vi "Create Connect Messages.vi"(8 "error in (no error)":errorcluster, 11 "Engine Data in":T2) -> (0 "error out":errorcluster, 1 "Connect Messages":T1[](array[typedef]), 2 "Disconnect Messages":T1[](array[typedef]), 3 "Engine Data out":T2)   [LabVIEW 2017, in "Routing and Faulting Engine.lvlib"]
uses:
  Routing and Faulting Engine.lvlib
  Engine Data.ctl
  Includes/CDMessaging.lvlibp/Producer/Abstract Producer/Abstract Producer.lvclass
  Shared/Compiled.Settings.ctl
  Shared/Communication Configuration.ctl
  Shared/Routing and Faulting Configuration.ctl
  Shared/Routing Channel Configuration.ctl
  Shared/Value-Connections Map.ctl
  Shared/Connection.ctl
  Shared/Alias Mapping.ctl
  Shared/FIFO Indices.ctl
  Device Inputs.ctl
  Device Outputs.ctl
  Producer Message.ctl
  Includes/CDMessaging.lvlibp/Message/Abstract Message/Abstract Message.lvclass
  f117cfd3-3adc-40fc-b63f-36de5ebdde45.vi
  3305a376-d4c0-444a-b726-8088d0367693.vi
  Shared/Routing and Faulting Shared.lvlib
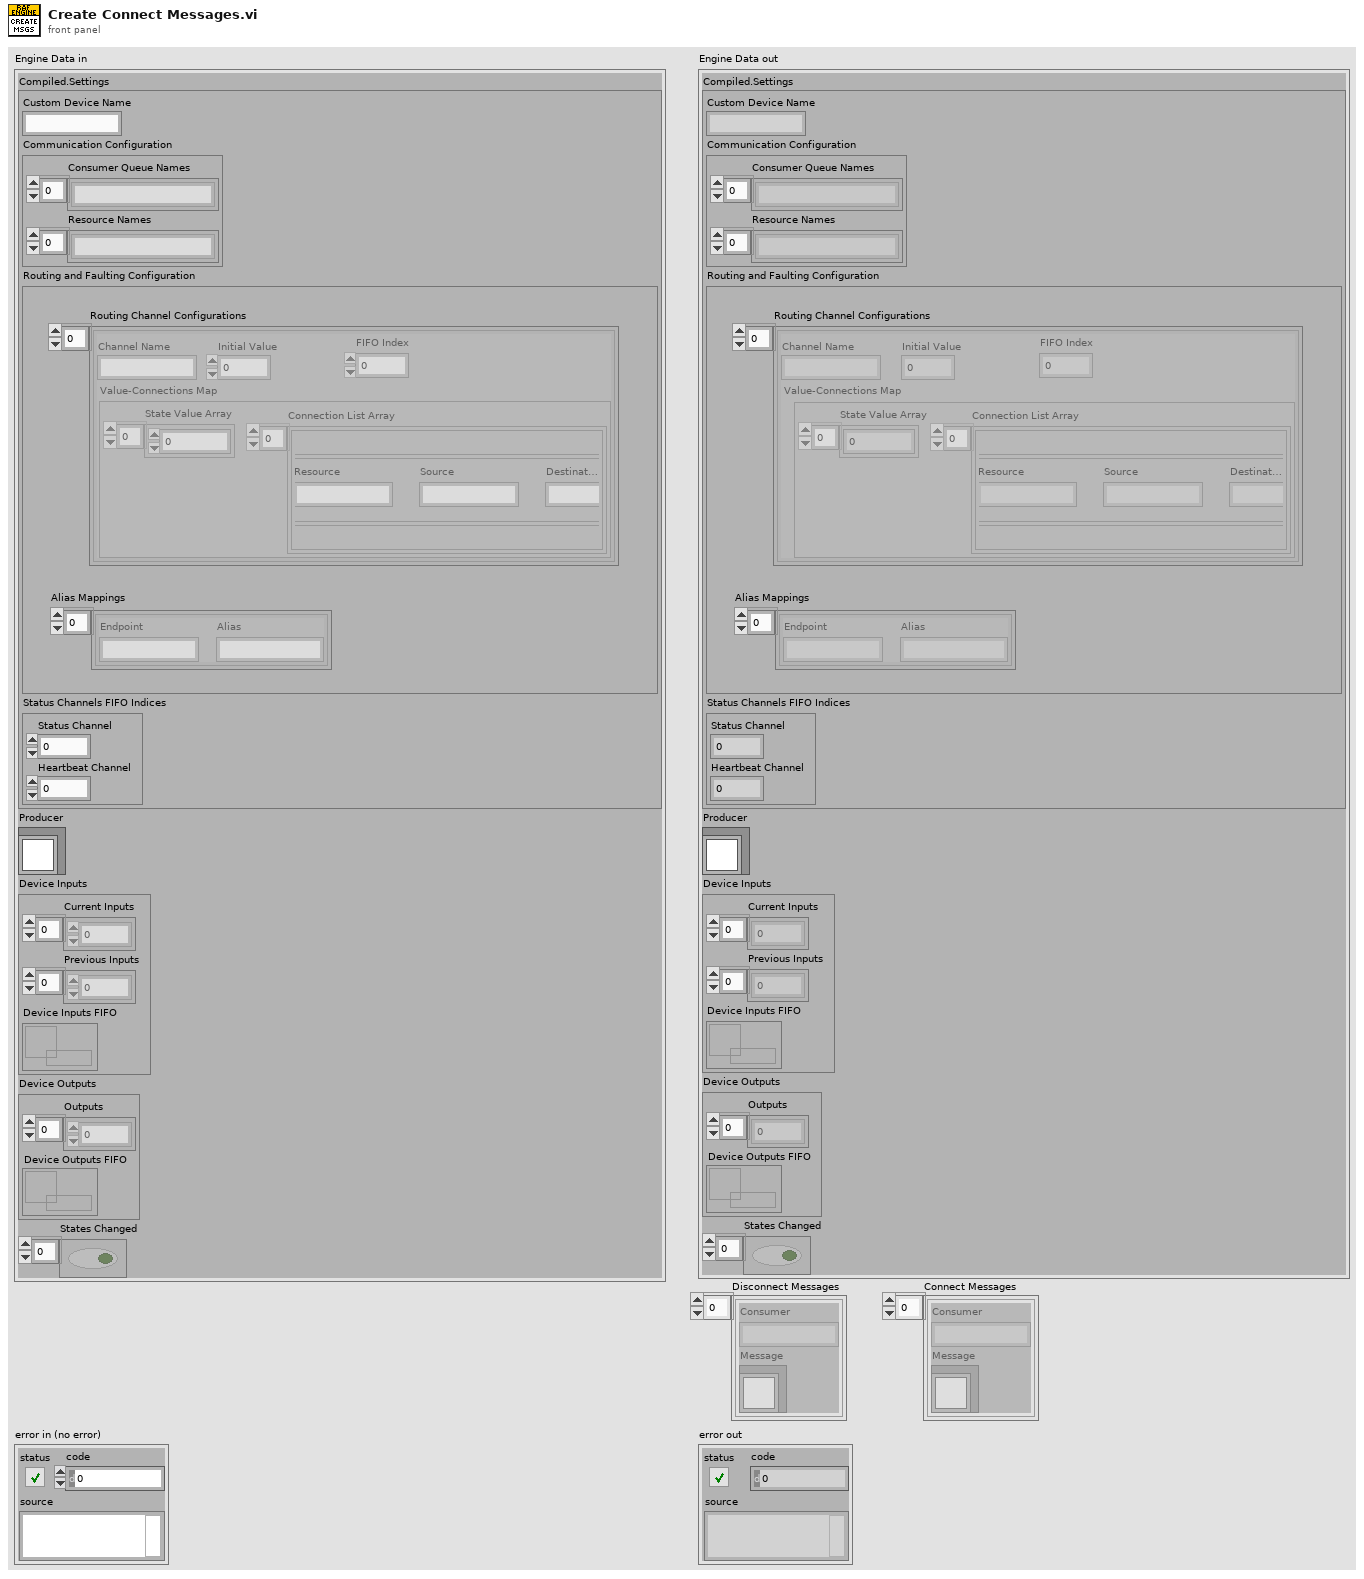
[diagram p1: front panel]
types:
  T1 = typedef "Routing and Faulting Engine.lvlib/Producer Message.ctl" = cluster{"Consumer":string, "Message":refnum<class "Abstract Message.lvclass">}
  T2 = typedef "Routing and Faulting Engine.lvlib/Engine Data.ctl" = cluster{"Compiled.Settings":T3, "Producer":refnum<class "Abstract Producer.lvclass">, "Device Inputs":T11, "Device Outputs":T12, "States Changed":bool[]}
  T3 = typedef "Routing and Faulting Shared.lvlib/Compiled.Settings.ctl" = cluster{"Custom Device Name":string, "Communication Configuration":T4, "Routing and Faulting Configuration":T5, "Status Channels FIFO Indices":T10}
  T4 = typedef "Routing and Faulting Shared.lvlib/Communication Configuration.ctl" = cluster{"Consumer Queue Names":string[], "Resource Names":string[]}
  T5 = typedef "Routing and Faulting Shared.lvlib/Routing and Faulting Configuration.ctl" = cluster{"Routing Channel Configurations":T6[], "Alias Mappings":T9[]}
  T6 = typedef "Routing and Faulting Shared.lvlib/Routing Channel Configuration.ctl" = cluster{"Channel Name":string, "Initial Value":dbl, "FIFO Index":i32, "Value-Connections Map":T7}
  T7 = typedef "Routing and Faulting Shared.lvlib/Value-Connections Map.ctl" = cluster{"State Value Array":i32[], "Connection List Array":cluster{"Connection List":T8[]}[]}
  T8 = typedef "Routing and Faulting Shared.lvlib/Connection.ctl" = cluster{"Resource":string, "Source":string, "Destination":string}
  T9 = typedef "Routing and Faulting Shared.lvlib/Alias Mapping.ctl" = cluster{"Endpoint":string, "Alias":string}
  T10 = typedef "Routing and Faulting Shared.lvlib/FIFO Indices.ctl" = cluster{"Status Channel":i32, "Heartbeat Channel":i32}
  T11 = typedef "Routing and Faulting Engine.lvlib/Device Inputs.ctl" = cluster{"Current Inputs":dbl[], "Previous Inputs":dbl[], "Device Inputs FIFO":refnum<k33>}
  T12 = typedef "Routing and Faulting Engine.lvlib/Device Outputs.ctl" = cluster{"Outputs":dbl[], "Device Outputs FIFO":refnum<k33>}
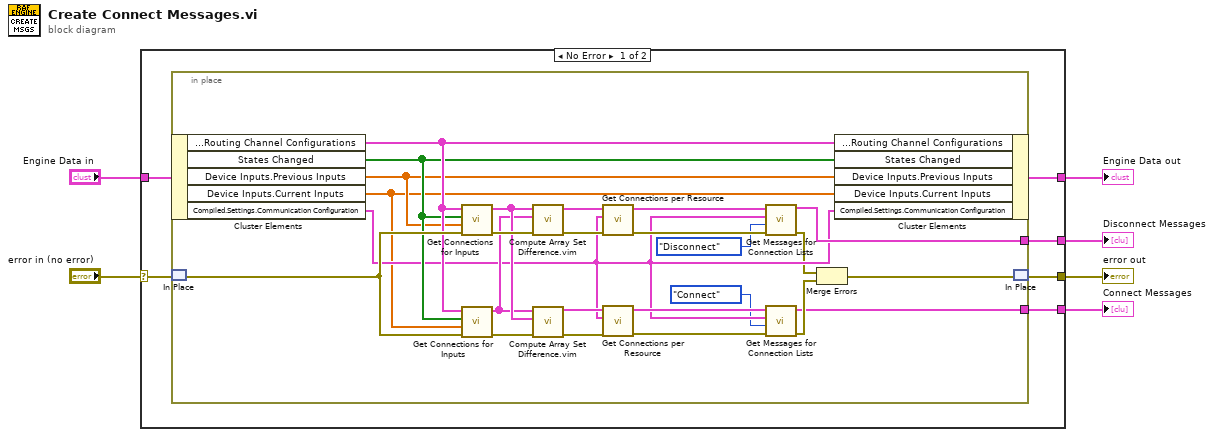
[diagram p0: block diagram]
diagram:
  n1 = case shown="No Error" "error in (no error)" {
    selector: "error in (no error)" -> [w12 w39]
    tunnel: "Engine Data in" -> [w8 w38]
    tunnel: [w11 w39] -> w4
    tunnel: [w10 w38] -> w3
    tunnel: [w9 _] -> w2
    tunnel: [w7 _] -> w1
    frame No Error {
      n2 = in-place {
        in-place-border: [w36] -> w9
        in-place-border: [w13] -> w7
        n3 = in-place-cluster #1(w8) -> ("Compiled.Settings.Routing and Faulting Configuration.Routing Channel Configurations"=w32:T6[], "States Changed"=w31:bool[], "Device Inputs.Previous Inputs"=w19:dbl[], "Device Inputs.Current Inputs"=w18:dbl[], "Compiled.Settings.Communication Configuration"=w21:T4)
        n4 = in-place-match #2(w12) -> (w33:errorcluster)
        n5 = call "Get Connections for Inputs.vi"("error in (no error)"=w33, "Inputs"=w19, "States Changed"=w31, "Routing Channel Configurations"=w32) -> ("error out"=w37:errorcluster, "Connection List"=w30:T8[])  [unwired: 6 in]
        n6 = call "Get Connections for Inputs.vi"("error in (no error)"=w33, "Inputs"=w18, "States Changed"=w31, "Routing Channel Configurations"=w32) -> ("error out"=w27:errorcluster, "Connection List"=w29:T8[])  [unwired: 6 in]
        n7 = call "Compute Array Set Difference.vim"("error in (no error)"=w37, "B"=w29, "A"=w30) -> ("error out"=w28:errorcluster, "A - B"=w26:T8[])  [unwired: 7 in]
        n8 = call "Compute Array Set Difference.vim"("error in (no error)"=w27, "B"=w30, "A"=w29) -> ("error out"=w23:errorcluster, "A - B"=w22:T8[])  [unwired: 7 in]
        n9 = call "Get Connections per Resource.vi"("error in (no error)"=w28, "Communication Configuration"=w21, "Connection List"=w26) -> ("error out"=w34:errorcluster, "Connection Lists for each Resource"=w35:cluster{T8[]}[])  [unwired: 7 in]
        n10 = call "Get Connections per Resource.vi"("error in (no error)"=w23, "Communication Configuration"=w21, "Connection List"=w22) -> ("error out"=w25:errorcluster, "Connection Lists for each Resource"=w24:cluster{T8[]}[])  [unwired: 7 in]
        n11 = call "Get Messages for Connection Lists.vi"("error in (no error)"=w34, "Message Type"=enum16{"Connect", "Disconnect"}."Disconnect", "Communication Configuration"=w21, "Connection Lists for each Resource"=w35) -> ("error out"=w17:errorcluster, "Messages"=w36:T1[])  [unwired: 6 in]
        n12 = call "Get Messages for Connection Lists.vi"("error in (no error)"=w25, "Message Type"=enum16{"Connect", "Disconnect"}."Connect", "Communication Configuration"=w21, "Connection Lists for each Resource"=w24) -> ("error out"=w16:errorcluster, "Messages"=w13:T1[])  [unwired: 6 in]
        n13 = Merge Errors(w17, w16) -> (w15:errorcluster)
        n14 = in-place-cluster #1("Compiled.Settings.Routing and Faulting Configuration.Routing Channel Configurations"=w32, "States Changed"=w31, "Device Inputs.Previous Inputs"=w19, "Device Inputs.Current Inputs"=w18, "Compiled.Settings.Communication Configuration"=w21) -> (w10:T2)
        n15 = in-place-match #2(w15) -> (w11:errorcluster)
      }
    }
    frame Error {
    }
  }
  "Engine Data out" <- w3
  "error out" <- w4
  "Disconnect Messages" <- w2
  "Connect Messages" <- w1
